vi "SQLite to JSON.vi"() -> ()   [LabVIEW 2020, in "CDM-Config.lvlib"]
uses:
  CDM-Config.lvlib
  Config-Sqlite/Config-Sqlite.lvclass
  C:/dev/lv20CE/lv-cdm/CDM-Config/Config Storage/Config Storage.lvclass
  Config-JSON/Config-JSON.lvclass
  Config Storage/Config Storage.lvclass
panel:
  out "error out":errorcluster
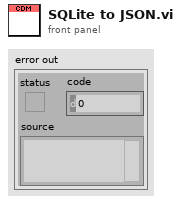
[diagram p1: front panel]
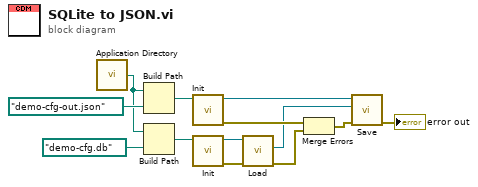
[diagram p0: block diagram]
diagram:
  n1 = call <vilib>:"Application Directory.vi"() -> ("Application Directory"=w11:path)
  n2 = Build Path(base path=w11, name or relative path=path "demo-cfg-out.json") -> (appended path=w9:path)
  n3 = Build Path(base path=w11, name or relative path=path "demo-cfg.db") -> (appended path=w10:path)
  n4 = call "Init.vi"("Path"=w9) -> ("error out"=w5:errorcluster, "Config-JSON out"=w6:refnum<class "Config-JSON.lvclass">)  [unwired: 9 in]
  n5 = call "Init.vi"("DB Path"=w10) -> ("error out"=w7:errorcluster, "Config-Sqlite out"=w8:refnum<class "Config-Sqlite.lvclass">)  [unwired: 9 in]
  n6 = call "Load.vi"("error in (no error)"=w7, "Config Storage in"=w8) -> ("error out"=w2:errorcluster, "Config"=w4:refnum<class "Config Manager.lvclass">)  [unwired: 7 in, 1 out]
  n7 = Merge Errors(w5, w2) -> (w3:errorcluster)
  n8 = call "Save.vi"("error in (no error)"=w3, "Config"=w4, "Config Storage in"=w6) -> ("error out"=→"error out":errorcluster)  [unwired: 7 in, 1 out]
